vi "Main Glb.vi"() -> ()   [LabVIEW 2019, in "Commonly VI.lvlib"]
uses:
  Commonly VI.lvlib
  Class/Main Process Class/Main Class.lvclass
panel:
  in  "S8 Barcode ID":string
  in  "Picture Path":path
  out "手動觸發AI站":bool
  out "Count Achieve":bool caption="元件使用次數"
  out "ArrivePercentage100":bool[](array[boolean])
  out "Percentage 80":bool[](array[boolean])
  out "工單資訊更新":bool
  in  "工單生產總數":string
  in  "Work No":string caption="工單號碼"
  out "Work No List path":path
  out "work no list":T1
  in  "Operator":string
  in  "品名":string
  in  "產品料號":string
  in  "工單號碼":string
  out "Input Registers400-499":u16[](array[numeric])
  out "Input Registers300-399":u16[](array[numeric])
  in  "S11 Table Scan ID":string
  in  "S4 Scan ID":string
  in  "熱熔 Barcode ID":string
  in  "熱熔 Tary ID":string
  in  "焊接 Barcode ID":string
  in  "焊接 Tary ID":string
  in  "S11 Barcode ID":string
  in  "S11 Tary ID":string
  in  "S4 Tary ID":string
  in  "S4 Barcode ID":string
  in  "S3 Barcode ID":string
  in  "S3 Tary ID":string
  in  "S2 Tary ID":string
  in  "S2 Barcode ID":string
  in  "Barcode ID":string
  out "ToolStringOut_Initial":string
  out "ToolStringOut_Program":string
  out "ToolStringOut_Format":string
  out "ToolStringOut_Scan":string
  out "Input Registers200-299":u16[](array[numeric])
  out "PLC MobsRegisters":u16[](array[numeric])
  out "Input Registers100-199":u16[](array[numeric])
  in  "Barcode Array":string[](array[string])
  in  "Tary ID":string
  in  "CurrentDataI":i32
  in  "CurrentDataF":dbl
  out "ModbusDataReadOK":bool
  out "Discrete Inputs":bool[](array[boolean])
  out "Input Registers0-99":u16[](array[numeric])
  out "ModbusInitialOK":bool
  out "ModbusSSOK":bool
  out "Modbus Status":string
  out "modbus error out":errorcluster
  out "ModbusQue":refnum<queue>
  out "Main Process Class":refnum<class "Main Class.lvclass">
  in  "Action":refnum<vi>
  in  "Axis Speed":refnum<vi>
  in  "ProjectRef":refnum<vi>
  in  "Operator Ref":refnum<vi>
  in  "System Path":path=path "C:/Users/Public/Documents/Vicomm"
  in  "Main Direction":string
  # "預防保養的部分"
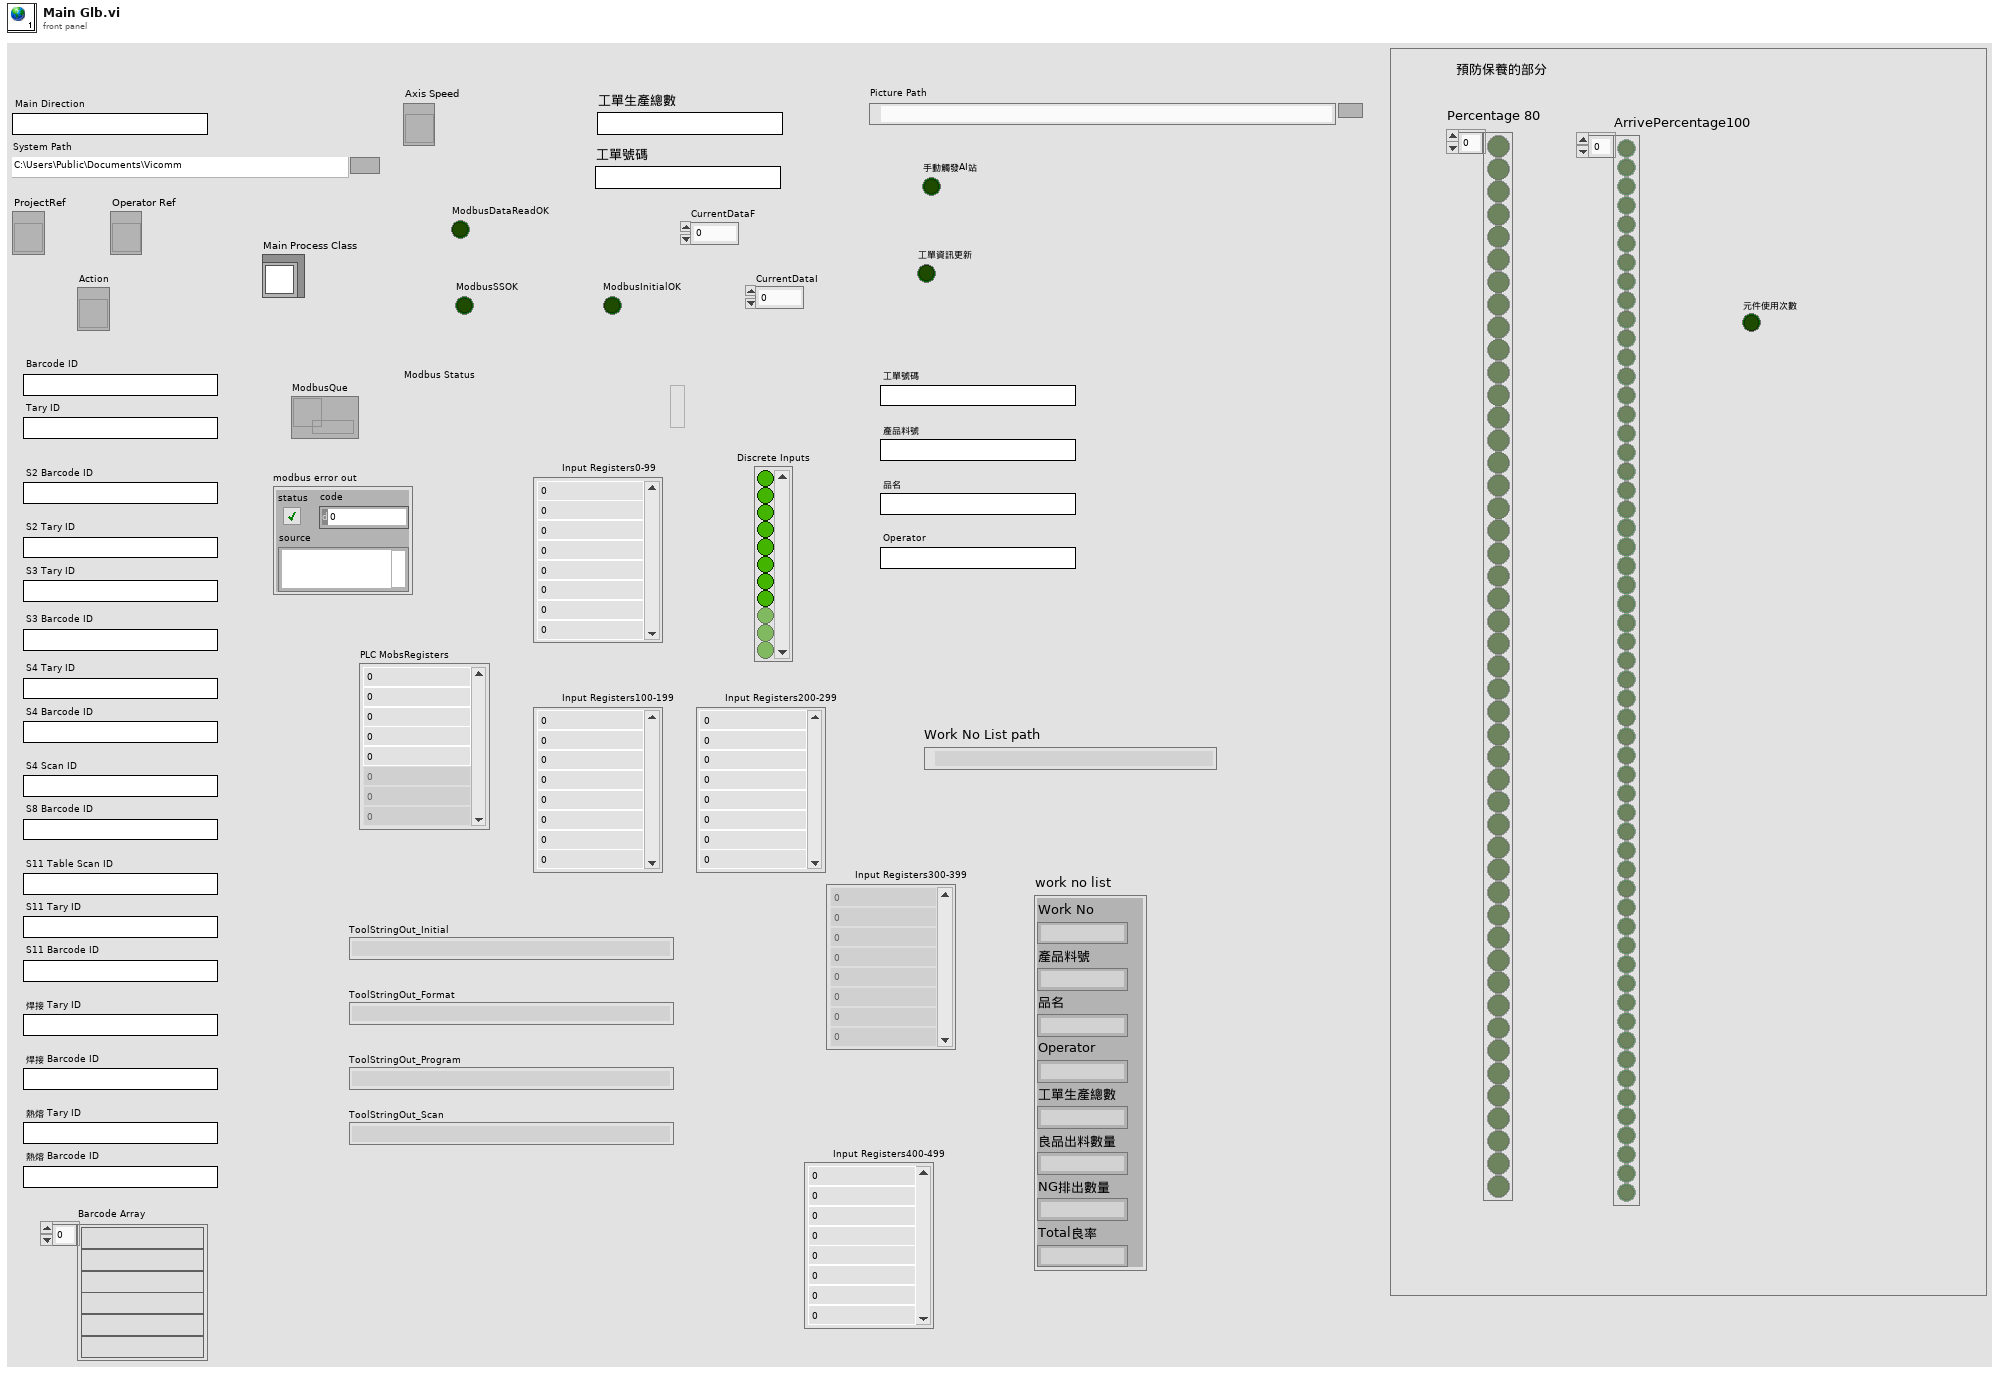
[diagram p1: front panel]
types:
  T1 = cluster{"Work No":string, "產品料號":string, "品名":string, "Operator":string, "工單生產總數":string, "良品出料數量":string, "NG排出數量":string, "Total良率":string}
diagram:
